vi "Update DOM XML Object.vi"(6 "Write to File?":bool, 7 "XML File Path":path, 8 "error in (no error)":errorcluster, 9 "New Value (String)":string, 10 "XPath expression to node":string, 11 "DOM Refnum (XML Document)":refnum<k20>) -> (0 "error out":errorcluster, 3 "XML string out":string)   [LabVIEW 2012]
doc: "SciScan 1.2 160622"
uses:
  <resource>/objmgr/DOMUserDefRef.rc
  <vilib>/xml/NI_XML.lvlib
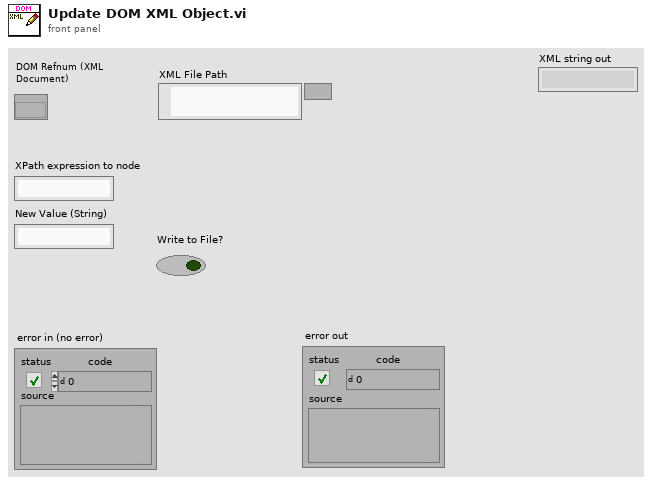
[diagram p1: front panel]
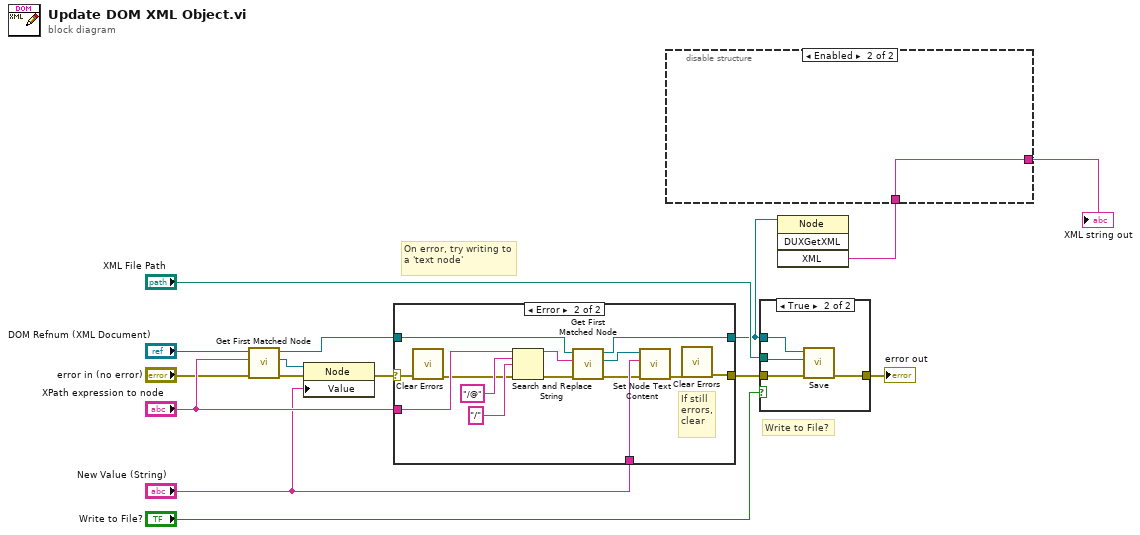
[diagram p0: block diagram]
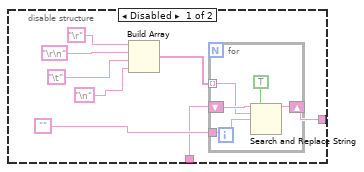
[diagram p2: hidden frame]
diagram:
  # "Write to File?"
  # "On error, try writing to a 'text node'"
  n1 = call <vilib>:"Get First Matched Node.vi"("error in (no error)"="error in (no error)", "XPath expression"="XPath expression to node", "node in"="DOM Refnum (XML Document)") -> ("error out"=w15:errorcluster, "node result"=w13:refnum<k20>, "node out"=w12:refnum<k20>)  [unwired: 6 in]
  n2 = property class="Node"(reference=w13, error in=w15, "Value"="New Value (String)") -> (error out=w14:errorcluster)  [unwired: 1 out]
  n3 = case shown="Error" w14 {
    selector: w14 -> [w17 w31]
    tunnel: [w17 w18] -> w6
    tunnel: "XPath expression to node" -> [_ w24]
    tunnel: w12 -> [w16 w30]
    tunnel: "New Value (String)" -> [_ w28]
    tunnel: [w16 w20] -> w3
    frame No Error {
    }
    frame Error {
      # "If still\nerrors,\nclear"
      n4 = call <vilib>:"Clear Errors.vi"("error in (no error)"=w31) -> ("error out"=w21:errorcluster)  [unwired: 6 in]
      n5 = Search and Replace String(input string=w24, search string="/@", replace string="/" ("replace string (\"\")"), error in=w21) -> (result string=w23:string, error out=w22:errorcluster)  [unwired: 4 in, 2 out]
      n6 = call <vilib>:"Get First Matched Node.vi"("error in (no error)"=w22, "XPath expression"=w23, "node in"=w30) -> ("error out"=w27:errorcluster, "node result"=w29:refnum<k20>, "node out"=w20:refnum<k20>)  [unwired: 6 in]
      n7 = call "Set Node Text Content.vi"("error in (no error)"=w27, "newValue"=w28, "node in"=w29) -> ("error out"=w19:errorcluster)  [unwired: 6 in, 2 out]
      n8 = call <vilib>:"Clear Errors.vi"("error in (no error)"=w19) -> ("error out"=w18:errorcluster)  [unwired: 6 in]
    }
  }
  n9 = case shown="True" "Write to File?" {
    tunnel: "XML File Path" -> [_ w36]
    tunnel: w6 -> [w32 w35]
    tunnel: w3 -> [_ w34]
    tunnel: [w32 w33] -> w5
    frame False {
    }
    frame True {
      n10 = call <vilib>:"Save.vi"("error in (no error)"=w35, "XML file path"=w36, "DOM document in"=w34) -> ("error out"=w33:errorcluster)  [unwired: 6 in, 2 out]
    }
  }
  "error out" <- w5
  n11 = invoke class="Node" method="DUXGetXML"(reference=w3) -> ("XML"=w1:string)  [unwired: 3 in, 3 out]
  n12 = disable-structure shown="Enabled" {
    disable-tunnel: [w43 w50] -> w2
    disable-tunnel: w1 -> [w42 w50]
    frame Disabled {
      n13 = Build Array("\r", "\r\n", "\t", "\n") -> (w39:string[])
      n14 = for {
        tunnel: "" ("replace string (\"\")") -> [w48]
        shift-right: [w47] -> w43
        shift-left: w42 -> [w46]
        tunnel: w39 -> [w45] mode=indexing
        n15 = Search and Replace String(replace all?=TRUE ("replace all? (F)"), input string=w46, search string=w45, replace string=w48) -> (result string=w47:string)  [unwired: 4 in, 3 out]
      }
    }
    frame Enabled {
    }
  }
  "XML string out" <- w2
